vi "Type Panel.vi"(11 "BooleanPanel in":refnum<class "BooleanPanel.lvclass">) -> ()   [LabVIEW 2020, in "Conditum-Tools.lvlib" / "BooleanPanel.lvclass"]
uses:
  BooleanPanel.lvclass
  C:/dev/lv20CE/lv-conditum-tools/Conditum-Tools/ColumnPanel/ColumnPanel.lvclass
  Conditum-Clone/Columns/Boolean/Boolean.lvclass
  BooleanPanel.lvclass/BooleanPanel.ctl
  ColumnPanel/ColumnPanel.lvclass
panel:
  in  "Default":bool
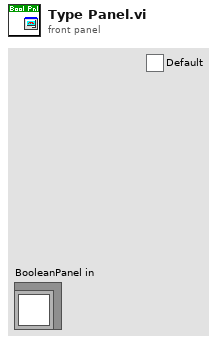
[diagram p1: front panel]
types:
  T1 = typedef "Conditum-Tools.lvlib/ColumnPanel.lvclass/Type Panel Event Reg.ctl" = refnum<event-registration>
  T2 = typedef "Conditu2.lvlib/Columns.lvlib/Boolean.lvclass/Definition.ctl" = cluster{"Default":bool}
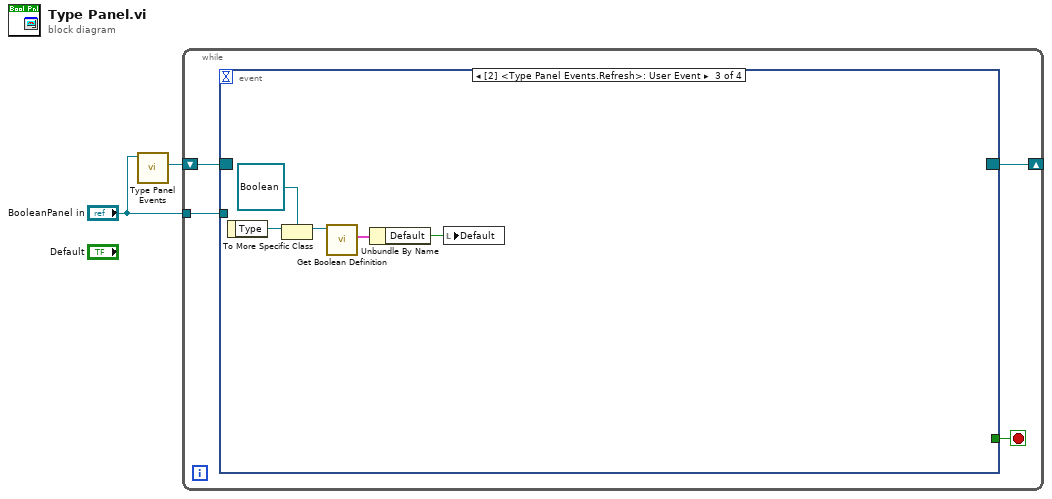
[diagram p0: block diagram]
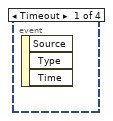
[diagram p2: hidden frame]
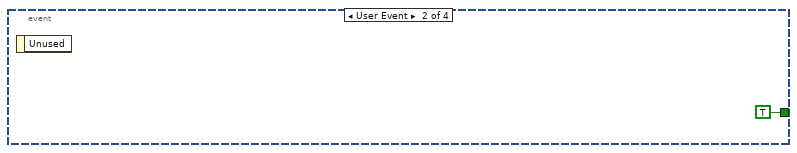
[diagram p3: hidden frame]
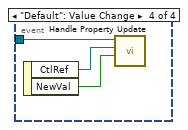
[diagram p4: hidden frame]
diagram:
  n1 = call "Type Panel Events.vi"("ColumnPanel"="BooleanPanel in") -> ("Type Panel Event Reg"=w1:T1)  [unwired: 10 in]
  n2 = while {
    tunnel: "BooleanPanel in" -> [w5]
    shift-right: [w3] -> _
    shift-left: w1 -> [w4]
    stop <- w6 stop-if-true
    n3 = event shown="[2] <Type Panel Events.Refresh>: User Event" {
      selector: w4 -> [_ _ _ _]
      dyn-events: [_ _ _ _] -> w3
      timeout: _ -> [_ _ _ _]
      tunnel: [_ TRUE _ _] -> w6
      tunnel: w5 -> [_ _ _ w15]
      event Timeout {
        n4 = event-data() -> ()  [unwired: 1 in, 3 out]
      }
      event User Event {
        n5 = event-data() -> ()  [unwired: 1 in, 1 out]
      }
      event User Event {
        n6 = event-data() -> ("Type"=w12:refnum<class "Type.lvclass">)  [unwired: 1 in]
        n7 = To More Specific Class(target class=refnum<class "Boolean.lvclass"> refnum ("Boolean"), reference=w12) -> (specific class reference=w9:refnum<class "Boolean.lvclass">)  [unwired: 1 in, 1 out]
        n8 = call "Get Boolean Definition.vi"("Boolean in"=w9) -> ("Definition"=w8:T2)  [unwired: 10 in]
        n9 = Unbundle By Name(w8) -> ("Default"=w11:bool)
        n10 = local write "Default"(w11) -> ()
      }
      event "Default": Value Change {
        n11 = event-data() -> ("CtlRef"=w14:refnum<vi>, "NewVal"=w13:bool)  [unwired: 1 in]
        n12 = call "Handle Property Update.vi"("Value"=w13, "Control"=w14, "ColumnPanel in"=w15) -> ()  [unwired: 7 in, 2 out]
      }
    }
  }
